vi "FP Front most.vi"(8 "error in (no error)":errorcluster, 10 "FP Frontmost":bool=TRUE, 11 "Panel in":refnum<class "Panel.lvclass">) -> (0 "error out":errorcluster, 3 "Panel out":refnum<class "Panel.lvclass">)   [LabVIEW 2021, in "Panel.lvlib" / "Panel.lvclass"]
uses:
  Panel.lvclass
  Panel.lvclass/Panel.ctl
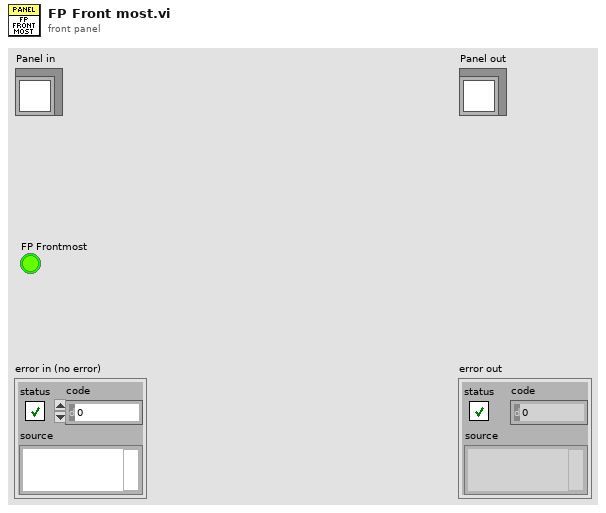
[diagram p1: front panel]
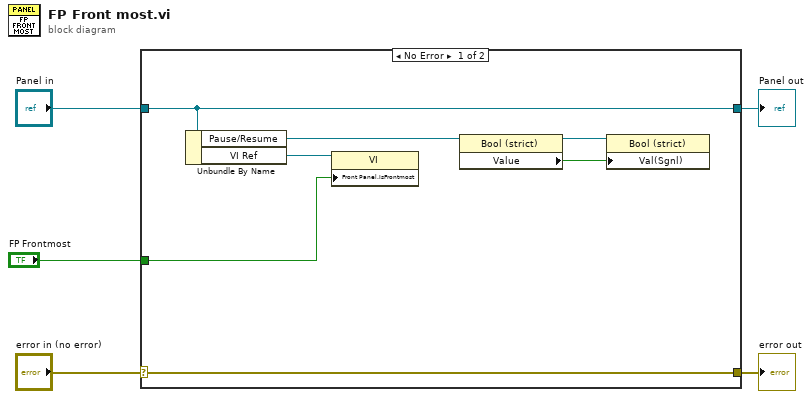
[diagram p0: block diagram]
diagram:
  n1 = case shown="No Error" "error in (no error)" {
    selector: "error in (no error)" -> [w12 w14]
    tunnel: [w12 w14] -> w4
    tunnel: [w11 w13] -> w2
    tunnel: "Panel in" -> [w11 w13]
    tunnel: "FP Frontmost" -> [w9 _]
    frame No Error {
      n2 = Unbundle By Name(w11) -> ("Pause/Resume"=w8:refnum<vi>, "VI Ref"=w10:refnum<vi>)
      n3 = property class="VI"(reference=w10, "Front Panel.IsFrontmost"=w9) -> ()  [unwired: 1 in, 2 out]
      n4 = property class="Bool (strict)"(reference=w8) -> (reference out=w7:refnum<vi>, "Value"=w6:bool)  [unwired: 1 in, 1 out]
      n5 = property class="Bool (strict)"(reference=w7, "Val(Sgnl)"=w6) -> ()  [unwired: 1 in, 2 out]
    }
    frame Error {
    }
  }
  "error out" <- w4
  "Panel out" <- w2
